vi "MS SQL UDL Path.vi"(1 "Bckup_DB?":bool) -> (0 "UDL File Location":path)   [LabVIEW 2020]
uses:
  <userlib>/_Controls/DB_State.ctl
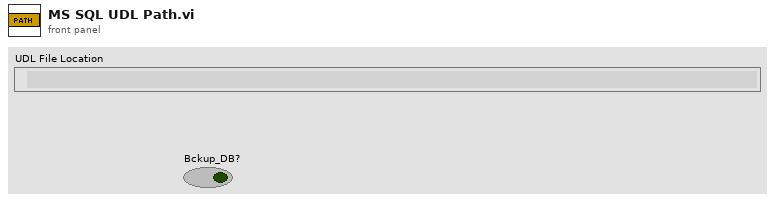
[diagram p1: front panel]
types:
  T1 = typedef "DB_State.ctl" = enum16{"Create DB", "Get DB"}
  T2 = cluster{"Data Path":path, "Calibration Path":path, "Settings Path":path, "Script Path":path, "DAQ Support":path, "Reporting Desktop":path, "Help":path}
  T3 = typedef "DB_ctrl.ctl" = cluster{"Calibration":path, "Parameter":path, "Script":path, "Help":path, "Password":path, "Database":path}
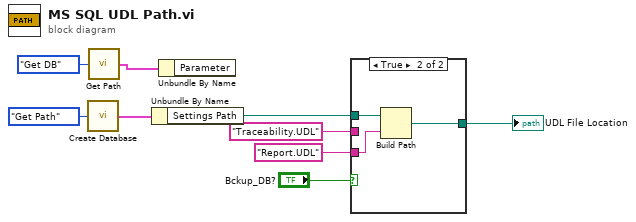
[diagram p0: block diagram]
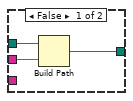
[diagram p2: hidden frame]
diagram:
  n1 = call <userlib>:"Create Database.vi"("Get/Create"=enum16{"Get Path", "Create Path"}."Get Path") -> ("Path Out"=w7:T2)  [unwired: 13 in, 1 out]
  n2 = call <userlib>:"Get Path.vi"("Get"=DB_State."Get DB") -> ("DB Paths"=w2:T3)  [unwired: 13 in, 1 out]
  n3 = Unbundle By Name(w7) -> ("Settings Path"=w1:path)
  n4 = Unbundle By Name(w2) -> ()  [unwired: 1 out]
  n5 = case shown="True" "Bckup_DB?" {
    tunnel: [w12 w15] -> w9
    tunnel: "Traceability.UDL" ("name or relative path") -> [w11 _]
    tunnel: w1 -> [w10 w14]
    tunnel: "Report.UDL" ("name or relative path") -> [_ w13]
    frame False {
      n6 = Build Path(base path=w10, name or relative path=w11) -> (appended path=w12:path)
    }
    frame True {
      n7 = Build Path(base path=w14, name or relative path=w13) -> (appended path=w15:path)
    }
  }
  "UDL File Location" <- w9
